vi "CHD_SIM_ENCODER_READ.vi"(11 "EncoderReference":T1) -> (2 "Distance":dbl, 6 "Velocity":dbl)   [LabVIEW 2019]
uses:
  <vilib>/Rock Robotics/WPI/Encoder/WPI_EncoderDevRef.ctl
  <vilib>/Rock Robotics/SystemInterfaces/Encoder/FPGA_EncoderIdx.ctl
  <vilib>/Rock Robotics/SystemInterfaces/Counter/FPGA_CounterCtrSystemIndex.ctl
  <vilib>/Rock Robotics/WPI/Encoder/WPI_EncoderType.ctl
  CHS_SIM_SIM_Globals.vi
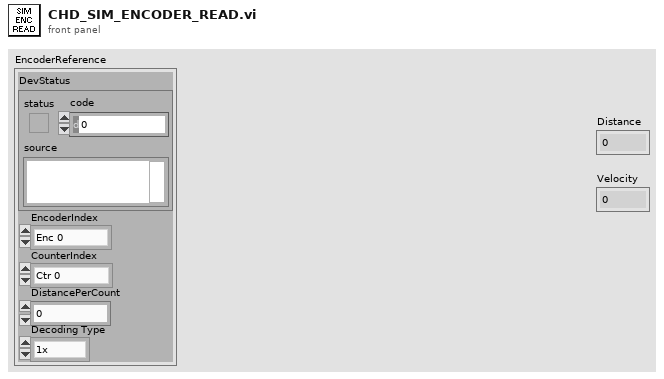
[diagram p1: front panel]
types:
  T1 = typedef "WPI_EncoderDevRef.ctl" = cluster{"DevStatus":errorcluster, "EncoderIndex":T2, "CounterIndex":T3, "DistancePerCount":dbl, "Decoding Type":T4}
  T2 = typedef "FPGA_EncoderIdx.ctl" = enum8{"Enc 0", "Enc 1", "Enc 2", "Enc 3", "Enc 4", "Enc 5", "Enc 6", "Enc 7", "Invalid"}
  T3 = typedef "FPGA_CounterCtrSystemIndex.ctl" = enum8{"Ctr 0", "Ctr 1", "Ctr 2", "Ctr 3", "Ctr 4", "Ctr 5", "Ctr 6", "Ctr 7", "Invalid"}
  T4 = typedef "WPI_EncoderType.ctl" = enum16{"1x", "2x", "4x"}
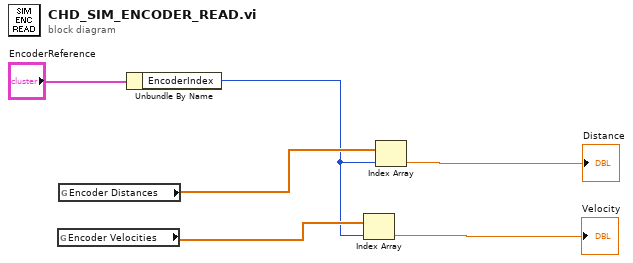
[diagram p0: block diagram]
diagram:
  n1 = global read "CHS_SIM_SIM_Globals.vi" "Encoder Velocities"() -> (w4:dbl[])
  n2 = global read "CHS_SIM_SIM_Globals.vi" "Encoder Distances"() -> (w5:dbl[])
  n3 = Unbundle By Name("EncoderReference") -> ("EncoderIndex"=w3:T2)
  n4 = Index Array(array=w4, index=w3) -> (element=→"Velocity":dbl)
  n5 = Index Array(array=w5, index=w3) -> (element=→"Distance":dbl)
